vi "Get Password From User.vi"(8 "error in":errorcluster, 11 "password":string="admin") -> (0 "error out":errorcluster, 3 "Success?":bool)   [LabVIEW 2015]
uses:
  <vilib>/event_ctls.llb/eventvkey.ctl
panel:
  in  "OK Button":bool
  in  "input":string
  # "Please Enter Password"
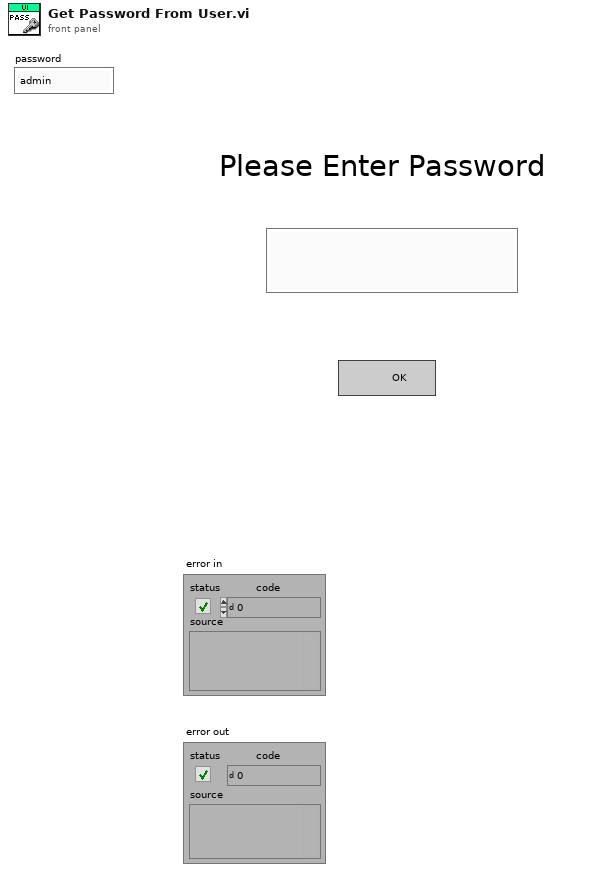
[diagram p1: front panel]
types:
  T1 = typedef "eventvkey.ctl" = enum16{"ASCII", "Enter", "Return", "Shift", "Ctrl", "Alt", "Cmd", "Opt", "Caps", "NumLock", "Clear", "Break", "Up", "Down", "Left", "Right", "Insert", "Delete", "Home", "End", "PageUp", "PageDown", "Escape", "Help", "Pause", "ScrollLock", "F1", "F2", "F3", "F4", "F5", "F6", "F7", "F8", "F9", "F10", "F11", "F12", "F13", "F14", "F15", "F16", "F17", "F18", "F19", "F20", "F21", "F22", "F23", "F24", "Play", "VolumeUp", "VolumeDown", "Mute", "Two Byte Char"}
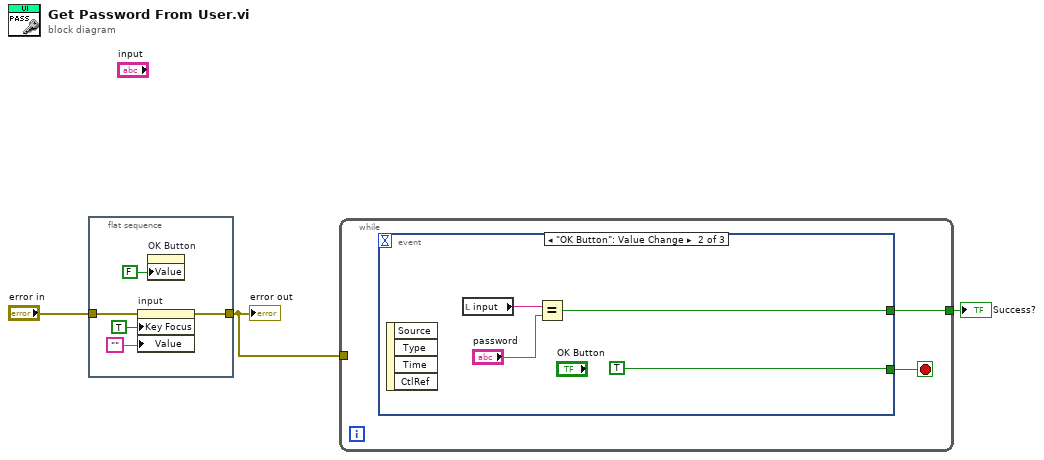
[diagram p0: block diagram]
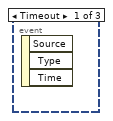
[diagram p2: hidden frame]
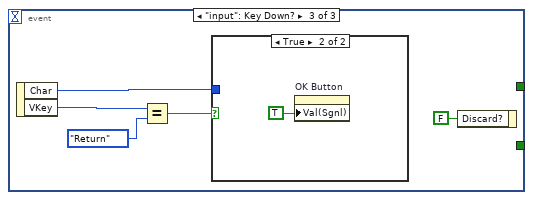
[diagram p3: hidden frame]
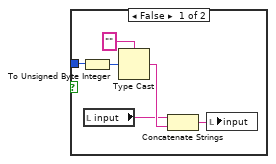
[diagram p4: hidden frame]
diagram:
  n1 = flat-sequence {
    tunnel: "error in" -> [w8]
    tunnel: [w7] -> w2
    frame #0 {
      n2 = property on="input" class="Str"(error in=w8, "Key Focus"=TRUE, "Value"="") -> (error out=w7:errorcluster)  [unwired: 1 in, 1 out]
      n3 = property on="OK Button" class="Bool (strict)"("Value"=FALSE ("OK Button")) -> ()  [unwired: 2 in, 2 out]
    }
  }
  n4 = while {
    tunnel: w2 -> [_]
    tunnel: [w9] -> w1
    stop <- w10 stop-if-true
    n5 = event shown="[1] \"OK Button\": Value Change" {
      selector: _ -> [_ _ _]
      dyn-events: _ -> [_ _ _]
      timeout: _ -> [_ _ _]
      tunnel: [_ TRUE ("OK Button") _] -> w10
      tunnel: [_ w13 _] -> w9
      event Timeout {
        n6 = event-data() -> ()  [unwired: 1 in, 3 out]
      }
      event "OK Button": Value Change {
        n7 = event-data() -> ()  [unwired: 1 in, 4 out]
        n8 = local read "input"() -> (w14:string)
        n9 = Equal?(x=w14, y="password") -> (x = y?=w13:bool)
      }
      event "input": Key Down? {
        n10 = event-data() -> ("Char"=w15:i16, "VKey"=w16:T1)  [unwired: 1 in]
        n11 = Equal?(x=w16, y=eventvkey."Return" ("x")) -> (x = y?=w18:bool)
        n12 = case shown="True" w18 {
          tunnel: w15 -> [w24 _]
          frame False {
            n13 = To Unsigned Byte Integer(number=w24) -> (unsigned 8bit integer=w25:u8)
            n14 = local read "input"() -> (w21:string)
            n15 = Type Cast(type="" ("input"), x=w25) -> (*(type *) &x=w22:string)
            n16 = Concatenate Strings(w21, w22) -> (w20:string)
            n17 = local write "input"(w20) -> ()
          }
          frame True {
            n18 = property on="OK Button" class="Bool (strict)"("Val(Sgnl)"=TRUE ("Value (Signaling)")) -> ()  [unwired: 2 in, 2 out]
          }
        }
        n19 = event-data("Discard?"=FALSE) -> ()  [unwired: 1 in, 1 out]
      }
    }
  }
  "Success?" <- w1
  "error out" <- w2
